vi "Constants.vi"() -> ()   [LabVIEW 2019, in "UDP Custom Device Shared.lvlib"]
doc: "Use this Global VI to access the GUIDs assigned to the page resources of the Custom Device."
uses:
  UDP Custom Device Shared.lvlib
panel:
  in  "Tab Control":enum32{"GUIDS", "Constants", "Properties"}(tab)=enum."Properties"
  in  "UDP Custom Device":string="076534e0-203a-4beb-b709-4fa362a5169d"
  in  "Destination Port":string="Destination Port"
  in  "Destination IP Address":string="Destination IP Address"
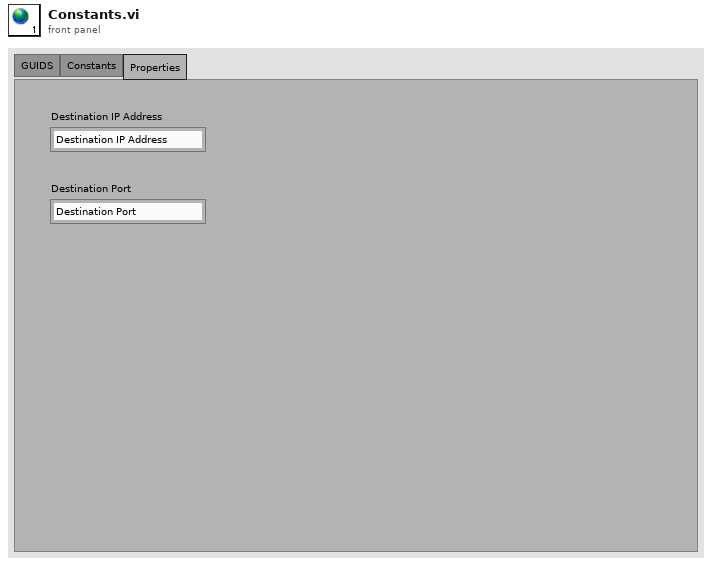
[diagram p1: front panel]
diagram:
